vi "8HP_AVmod_EnFlo_Specific.vi"(2 "Datalog file path (full)":path, 3 "COM port":refnum<visa-resource-name>, 4 "Log data stream":bool, 5 "Set data rate (Hz)":u8(ring)=14 items=["1", "2", "4", "5", "8", "10", "16", "20", "25", "32", "40", "50", "64", "80", "100", "125", "160", "200", "250", "320", "400", "500", "625", "800", "1000"], 6 "N samples":u32=1000, 7 "Command":T2="D") -> (0 "Error":errorcluster, 1 "All samples out":sgl[][](array[numeric]))   [LabVIEW 2020]
uses:
  ctls/8HP_Cmd (USB).ctl
  Globals/Meas_global.vi
panel:
  in  "Main":T1(tab)
  out "Serial number":sgl
  out "Subsystems ok":bool[](array[boolean])
  out "Pressure sensor values in range":bool[](array[boolean])
  out "Pressure sensor temperatures in range":bool[](array[boolean])
  out "Pressure sensor EEPROM checksums ok":bool[](array[boolean])
  out "P_raw_Azero":sgl[](array[numeric])
  out "n":u16
  out "Auto zero progBar":u16(slide) caption="Collecting samples, please maintain dP = 0" scale=0.0..1000.0
  in  "EEPROM array 2":u16[](array[numeric])
  in  "EEPROM array":sgl[](array[numeric])
  out "Chk ok":bool
  out "EEPROM Checksum":u16 format="%04x"
  out "received":bool
  out "Returned data rate (Hz)":u16
  out "sent":bool
  out "frm err":u32
  out "chk err":u32
  in  "Stop Data":bool
  out "Relative humidity (%)":sgl
  out "Env. sensor die temperature (deg C)":sgl
  out "External thermistor 0 temperature (deg C)":sgl
  out "Atmospheric pressure (mbar)":sgl
  out "Checksum ok":bool
  out "Gyration vector (deg / s)":sgl[](array[numeric])
  out "Acceleration vector (g)":sgl[](array[numeric])
  out "Pressures":sgl[][](graph)
  out "Stream enabled":bool
  out "External thermistor 1 temperature (deg C)":sgl
  # "Paul Nathan 05/2019"
  # "Output array order:\nP0 (Pa)\n  |\nP7 (Pa)\nT0 (deg C)\nT1 (deg C)\nP_atmos (mbar)\nT_env (deg C)\nRH (%)\nax (g)\nay (g)\naz (g)\nwx (deg / s)\nwy (deg / s)\nwz (deg / s)"
  # "Environmental sensor present"
  # "Inertial sensor present"
  # "Accelerometer self test pass"
  # "Gyroscope self test pass"
  # "External thermistor 0 value in range"
  # "External thermistor 1 value in range"
  # "MCU EEPROM checksum ok"
  # "Pressure sensor 0 value in range"
  # "Pressure sensor 1 value in range"
  # "Pressure sensor 2 value in range"
  # "Pressure sensor 3 value in range"
  # "Pressure sensor 4 value in range"
  # "Pressure sensor 5 value in range"
  # "Pressure sensor 6 value in range"
  # "Pressure sensor 7 value in range"
  # "Pressure sensor 0 temperature in range"
  # "Pressure sensor 1 temperature in range"
  # "Pressure sensor 2 temperature in range"
  # "Pressure sensor 3 temperature in range"
  # "Pressure sensor 4 temperature in range"
  # "Pressure sensor 5 temperature in range"
  # "Pressure sensor 6 temperature in range"
  # "Pressure sensor 7 temperature in range"
  # "Pressure sensor 0 EEPROM checksum okay"
  # "Pressure sensor 1 EEPROM checksum okay"
  # "Pressure sensor 2 EEPROM checksum okay"
  # "Pressure sensor 3 EEPROM checksum okay"
  # "Pressure sensor 4 EEPROM checksum okay"
  # "Pressure sensor 5 EEPROM checksum okay"
  # "Pressure sensor 6 EEPROM checksum okay"
  # "Pressure sensor 7 EEPROM checksum okay"
  # "of 1000"
  # "P0 raw auto-zero"
  # "P1 raw auto-zero"
  # "P2 raw auto-zero"
  # "P3 raw auto-zero"
  # "P4 raw auto-zero"
  # "P5 raw auto-zero"
  # "P6 raw auto-zero"
  # "P7 raw auto-zero"
  # "Power-up defaults"
  # "Data rate (Hz)"
  # "TTL streaming"
  # "USB streaming"
  # "TTL stream contains full data"
  # "Accelerometer range mode"
  # "Gyroscope range mode"
  # "IMU rate mode"
  # "P0 raw auto-zero"
  # "P1 raw auto-zero"
  # "P2 raw auto-zero"
  # "P3 raw auto-zero"
  # "P4 raw auto-zero"
  # "P5 raw auto-zero"
  # "P6 raw auto-zero"
  # "P7 raw auto-zero"
  # "Atmospheric pressure offset (Pa)"
  # "External thermistor 0 temperature offset (deg C)"
  # "External thermistor 1 temperature offset (deg C)"
  # "Serial number"
  # "Baud rate (bps)"
  # "Accelerometer vector magnitude scale factor"
  # "Gyroscope x component offset (deg / s)"
  # "Gyroscope y component offset (deg / s)"
  # "Gyroscope z component offset (deg / s)"
  # "w_x"
  # "w_y"
  # "w_z"
  # "a_x"
  # "a_y"
  # "a_z"
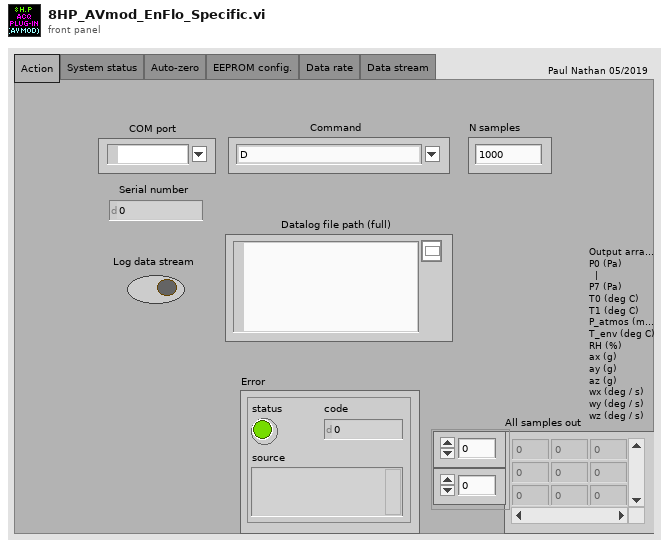
[diagram p1: front panel]
types:
  T1 = enum32{"Action", "System status", "Auto-zero", "EEPROM config.", "Data rate", "Data stream"}
  T2 = typedef "8HP_Cmd (USB).ctl" = string
  T3 = enum16{"open", "replace", "create", "open or create", "replace or create", "replace or create with confirmation"}
  T4 = typedef "Rendezvous RefNum" = refnum<k1>
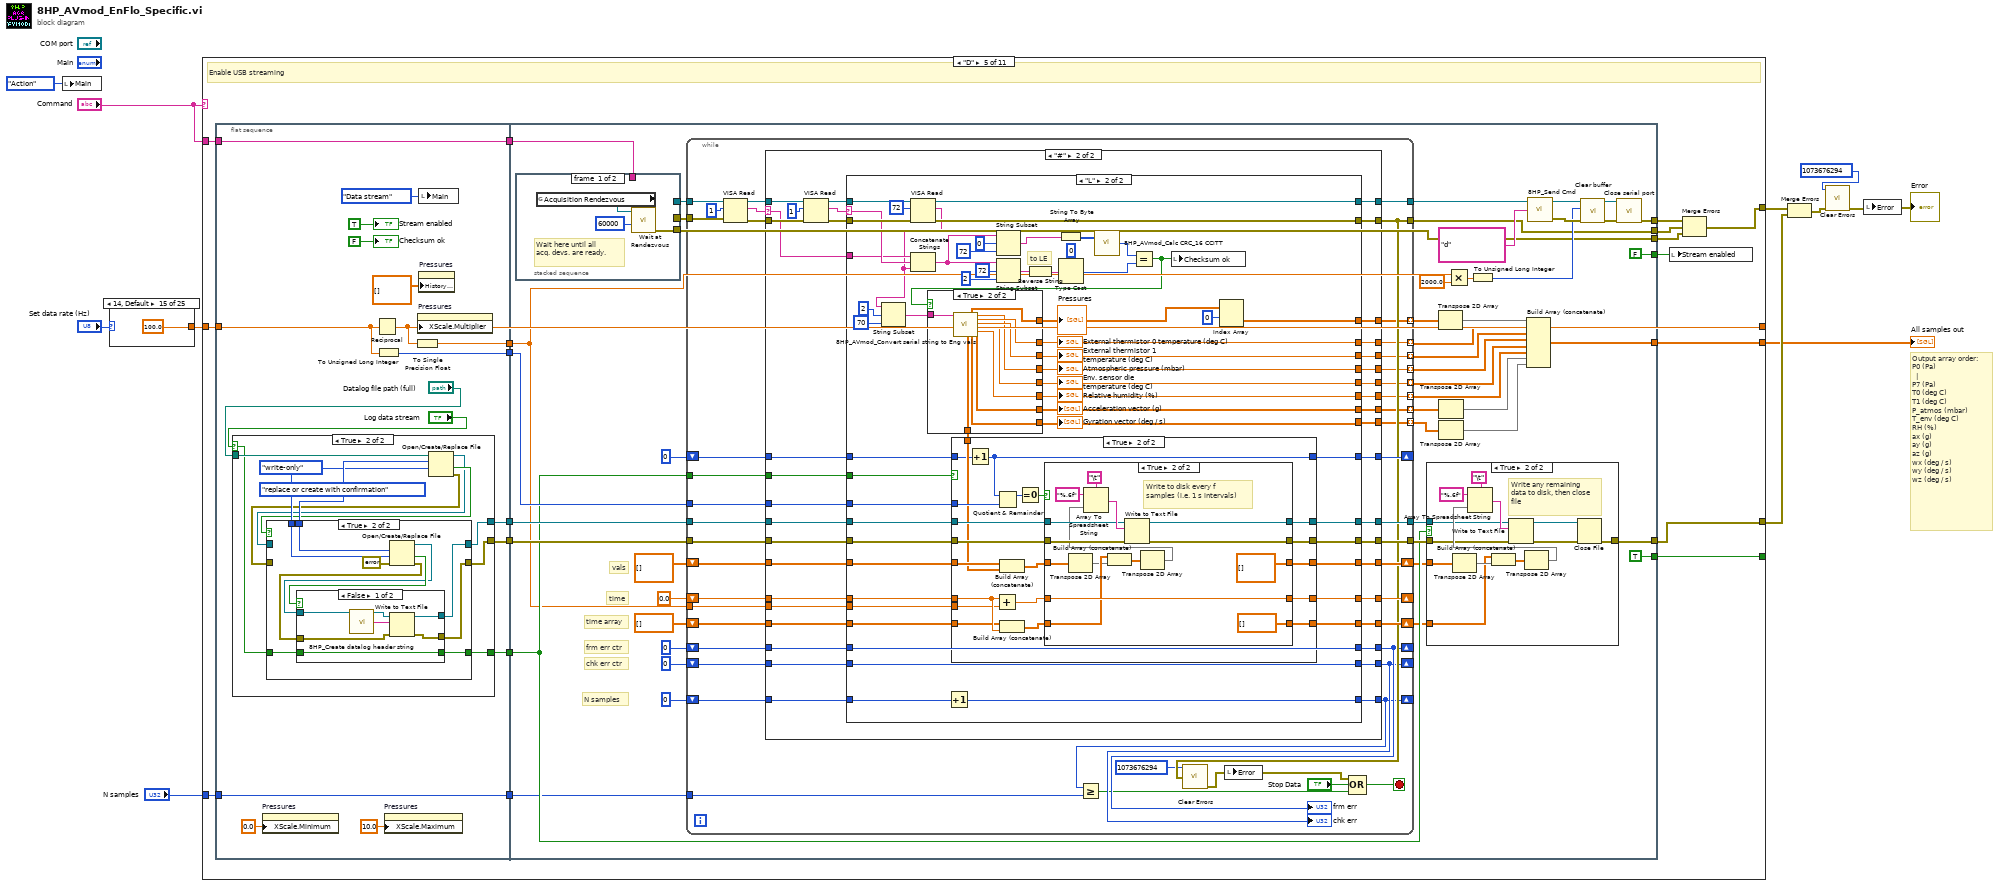
[diagram p0: block diagram]
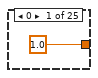
[diagram p2: hidden frame]
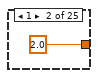
[diagram p3: hidden frame]
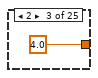
[diagram p4: hidden frame]
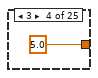
[diagram p5: hidden frame]
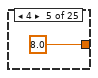
[diagram p6: hidden frame]
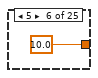
[diagram p7: hidden frame]
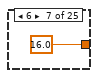
[diagram p8: hidden frame]
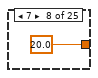
[diagram p9: hidden frame]
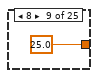
[diagram p10: hidden frame]
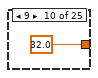
[diagram p11: hidden frame]
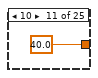
[diagram p12: hidden frame]
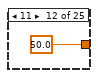
[diagram p13: hidden frame]
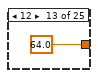
[diagram p14: hidden frame]
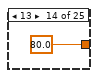
[diagram p15: hidden frame]
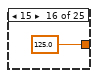
[diagram p16: hidden frame]
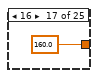
[diagram p17: hidden frame]
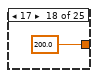
[diagram p18: hidden frame]
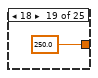
[diagram p19: hidden frame]
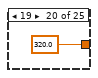
[diagram p20: hidden frame]
diagram:
  # "Output array order:\nP0 (Pa)\n  |\nP7 (Pa)\nT0 (deg C)\nT1 (deg C)\nP_atmos (mbar)\nT_env (deg C)\nRH (%)\nax (g)\nay (g)\naz (g)\nwx (deg / s)\nwy (deg / s)\nwz (deg / s)"
  n1 = local write "Main"(T1."Action" ("Main")) -> ()
  n2 = case shown="14, Default" "Set data rate (Hz)" {
    tunnel: [1.0 2.0 4.0 5.0 8.0 10.0 16.0 20.0 25.0 32.0 40.0 50.0 64.0 80.0 100.0 125.0 160.0 200.0 250.0 320.0 400.0 500.0 625.0 800.0 1000.0] -> w6
    frame 0 {
    }
    frame 1 {
    }
    frame 2 {
    }
    frame 3 {
    }
    frame 4 {
    }
    frame 5 {
    }
    frame 6 {
    }
    frame 7 {
    }
    frame 8 {
    }
    frame 9 {
    }
    frame 10 {
    }
    frame 11 {
    }
    frame 12 {
    }
    frame 13 {
    }
    frame 14, Default {
    }
    frame 15 {
    }
    frame 16 {
    }
    frame 17 {
    }
    frame 18 {
    }
    frame 19 {
    }
    frame 20 {
    }
    frame 21 {
    }
    frame 22 {
    }
    frame 23 {
    }
    frame 24 {
    }
  }
  n3 = case shown="\"D\"" "Command" {
    tunnel: [w41 w80 w117 w186 w277 w631 w655 w711 w747 FALSE FALSE] -> _
    tunnel: "Command" -> [w40 w79 w116 w197 w276 w633 w661 w717 w746 _ _]
    tunnel: [w38 w77 w114 w190 w264 w632 w656 w712 w744 errorcluster {"status"=FALSE, "code"=0, "source"=""} ("Error out") errorcluster {"status"=FALSE, "code"=0, "source"=""} ("Error out")] -> w10
    tunnel: [_ _ _ _ w274 _ _ _ _ _ _] -> w9
    tunnel: w6 -> [w37 w76 w113 w194 w267 w629 _ _ w743 w767 w770]
    tunnel: [w37 w76 w113 w194 w267 w629 w657 w713 w743 w767 w770] -> _
    tunnel: "N samples" -> [_ _ _ _ w262 _ _ _ _ _ _]
    tunnel: [_ _ _ _ w261 _ _ _ _ _ _] -> w3
    frame "S", "s" {
      # "Perform self-test and retrieve status bytes, Retrieve status bytes"
      n4 = flat-sequence {
        tunnel: w40 -> [w44]
        tunnel: [w44] -> w39
        tunnel: [TRUE] -> w41
        tunnel: w39 -> [w50]
        tunnel: [w45] -> w38
        frame #0 {
          w43 = bool[] [] ("Pressure sensor EEPROM checksums ok")
          n5 = local write "Main"(T1."System status" ("Main")) -> ()
          "Pressure sensor EEPROM checksums ok" <- w43
          "Pressure sensor temperatures in range" <- w43
          "Pressure sensor values in range" <- w43
          "Subsystems ok" <- w43
        }
        frame #1 {
          w55 = 1 ("length (rest)")
          w63 = u8 0 ("byte count")
          n6 = local read "COM port"() -> (w51:refnum<visa-resource-name>)
          n7 = call "Open serial port.vi"("timeout (ms)"=u32 5000, "VISA resource name"=w51) -> ("Error out"=w73:errorcluster, "VISA resource name out"=w74:refnum<visa-resource-name>)  [unwired: 8 in]
          n8 = call "8HP_Send Cmd.vi"("Error In"=w73, "Operation"=w50, "Port"=w74) -> ("Error Out"=w71:errorcluster, "Port out"=w72:refnum<visa-resource-name>)  [unwired: 1 in]
          n9 = VISA Read(VISA resource name=w72, byte count=u32 4, error in (no error)=w71) -> (VISA resource name out=w69:refnum<visa-resource-name>, read buffer=w58:string, error out=w68:errorcluster)  [unwired: 1 out]
          n10 = call "Close serial port.vi"("Error in"=w68, "VISA resource name"=w69) -> ("Error out"=w45:errorcluster)  [unwired: 9 in]
          n11 = String Subset(string=w58, offset (0)=0, length (rest)=w55) -> (substring=w67:string)
          n12 = String Subset(string=w58, offset (0)=1, length (rest)=w55) -> (substring=w66:string)
          n13 = String Subset(string=w58, offset (0)=2 ("length (rest)"), length (rest)=w55) -> (substring=w65:string)
          n14 = String Subset(string=w58, offset (0)=3, length (rest)=w55) -> (substring=w64:string)
          n15 = Type Cast(type=w63, x=w67) -> (*(type *) &x=w62:u8)
          n16 = Type Cast(type=w63, x=w66) -> (*(type *) &x=w61:u8)
          n17 = Type Cast(type=w63, x=w65) -> (*(type *) &x=w60:u8)
          n18 = Type Cast(type=w63, x=w64) -> (*(type *) &x=w59:u8)
          n19 = Number To Boolean Array(number=w62) -> (Boolean array=w49:bool[])
          n20 = Number To Boolean Array(number=w61) -> (Boolean array=w48:bool[])
          n21 = Number To Boolean Array(number=w60) -> (Boolean array=w47:bool[])
          n22 = Number To Boolean Array(number=w59) -> (Boolean array=w46:bool[])
          n23 = local write "Pressure sensor EEPROM checksums ok"(w49) -> ()
          n24 = local write "Pressure sensor temperatures in range"(w48) -> ()
          n25 = local write "Pressure sensor values in range"(w47) -> ()
          n26 = local write "Subsystems ok"(w46) -> ()
        }
      }
    }
    frame "Z", "z" {
      # "Perform permanent auto-zero (write values to EEPROM), Perform temporary auto-zero"
      n27 = flat-sequence {
        tunnel: w79 -> [w84]
        tunnel: [w84] -> w78
        tunnel: [TRUE] -> w80
        tunnel: w78 -> [w91]
        tunnel: [w87] -> w77
        frame #0 {
          n28 = local write "Main"(T1."Auto-zero" ("Main")) -> ()
          "P_raw_Azero" <- sgl[] [] ("P_raw_Azero")
          "Auto zero progBar" <- u16 0 ("Collecting samples, please maintain dP = 0")
        }
        frame #1 {
          n29 = local read "COM port"() -> (w92:refnum<visa-resource-name>)
          n30 = call "Open serial port.vi"("timeout (ms)"=u32 16000, "VISA resource name"=w92) -> ("Error out"=w99:errorcluster, "VISA resource name out"=w100:refnum<visa-resource-name>)  [unwired: 8 in]
          n31 = call "8HP_Send Cmd.vi"("Error In"=w99, "Operation"=w91, "Port"=w100) -> ("Error Out"=w97:errorcluster, "Port out"=w98:refnum<visa-resource-name>)  [unwired: 1 in]
          n32 = VISA Read(VISA resource name=w98, byte count=u32 32, error in (no error)=w97) -> (VISA resource name out=w95:refnum<visa-resource-name>, read buffer=w88:string, error out=w94:errorcluster)  [unwired: 1 out]
          n33 = for {
            N: 1000 -> [_]
            shift-right: [w102] -> _
            shift-left: u16 0 -> [w103]
            n34 = Increment(x=w103) -> (x+1=w102:u16)
            "n" <- w102
            n35 = Wait (ms)(milliseconds to wait=u32 10) -> ()  [unwired: 1 out]
            n36 = local write "Auto zero progBar"(w102) -> ()
          }
          n37 = for {
            N: 8 -> [_]
            tunnel: [w106] -> w90 mode=indexing
            tunnel: w88 -> [w105]
            i -> [w112]
            w110 = 4 ("x")
            # "to BE"
            n38 = Multiply(x=w110, y=w112) -> (x*y=w111:i32)
            n39 = String Subset(string=w105, offset (0)=w111, length (rest)=w110) -> (substring=w109:string)
            n40 = Reverse String(1:w109) -> (0:w108:string)
            n41 = Type Cast(type=sgl 0.0 ("byte count"), x=w108) -> (*(type *) &x=w106:sgl)
          }
          n42 = call "Close serial port.vi"("Error in"=w94, "VISA resource name"=w95) -> ("Error out"=w87:errorcluster)  [unwired: 9 in]
          n43 = local write "P_raw_Azero"(w90) -> ()
        }
      }
    }
    frame "R" {
      # "Read all EEPROM values"
      n44 = flat-sequence {
        tunnel: w116 -> [w121]
        tunnel: [w121] -> w115
        tunnel: [TRUE] -> w117
        tunnel: w115 -> [w159]
        tunnel: [w157] -> w114
        frame #0 {
          n45 = local write "EEPROM array"(sgl[] [] ("EEPROM array")) -> ()
          n46 = local write "EEPROM array 2"(u16[] [] ("EEPROM array 2")) -> ()
          n47 = local write "Main"(T1."EEPROM config." ("Main")) -> ()
        }
        frame #1 {
          # "to BE"
          # "to BE"
          n48 = local read "COM port"() -> (w160:refnum<visa-resource-name>)
          n49 = call "Open serial port.vi"("timeout (ms)"=u32 5000, "VISA resource name"=w160) -> ("Error out"=w167:errorcluster, "VISA resource name out"=w168:refnum<visa-resource-name>)  [unwired: 8 in]
          n50 = call "8HP_Send Cmd.vi"("Error In"=w167, "Operation"=w159, "Port"=w168) -> ("Error Out"=w165:errorcluster, "Port out"=w166:refnum<visa-resource-name>)  [unwired: 1 in]
          n51 = VISA Read(VISA resource name=w166, byte count=u32 78, error in (no error)=w165) -> (VISA resource name out=w163:refnum<visa-resource-name>, read buffer=w126:string, error out=w162:errorcluster)  [unwired: 1 out]
          n52 = call "Close serial port.vi"("Error in"=w162, "VISA resource name"=w163) -> ("Error out"=w157:errorcluster)  [unwired: 9 in]
          n53 = String Subset(string=w126, offset (0)=0, length (rest)=56 ("length (rest)")) -> (substring=w155:string)
          n54 = String Subset(string=w126, offset (0)=64, length (rest)=12 ("length (rest)")) -> (substring=w150:string)
          n55 = String Subset(string=w126, offset (0)=56, length (rest)=2 ("length (rest)")) -> (substring=w140:string)
          n56 = String Subset(string=w126, offset (0)=58, length (rest)=6 ("length (rest)")) -> (substring=w135:string)
          n57 = String Subset(string=w126, offset (0)=76, length (rest)=2 ("length (rest)")) -> (substring=w127:string)
          n58 = String Subset(string=w126, offset (0)=0, length (rest)=76 ("length (rest)")) -> (substring=w123:string)
          n59 = for {
            N: 14 -> [_]
            tunnel: [w181] -> w149 mode=indexing
            tunnel: w155 -> [w180]
            i -> [w185]
            w183 = 4 ("x")
            # "to BE"
            n60 = Multiply(x=w183, y=w185) -> (x*y=w184:i32)
            n61 = String Subset(string=w180, offset (0)=w184, length (rest)=w183) -> (substring=w179:string)
            n62 = Reverse String(1:w179) -> (0:w178:string)
            n63 = Type Cast(type=sgl 0.0 ("byte count"), x=w178) -> (*(type *) &x=w181:sgl)
          }
          n64 = for {
            N: 3 -> [_]
            tunnel: [w173] -> w148 mode=indexing
            tunnel: w150 -> [w172]
            i -> [w177]
            w175 = 4 ("x")
            # "to BE"
            n65 = Multiply(x=w175, y=w177) -> (x*y=w176:i32)
            n66 = String Subset(string=w172, offset (0)=w176, length (rest)=w175) -> (substring=w171:string)
            n67 = Reverse String(1:w171) -> (0:w170:string)
            n68 = Type Cast(type=sgl 0.0 ("byte count"), x=w170) -> (*(type *) &x=w173:sgl)
          }
          n69 = Reverse String(1:w140) -> (0:w146:string)
          n70 = Reverse String(1:w127) -> (0:w131:string)
          n71 = String To Byte Array(string=w123) -> (unsigned byte array=w134:u8[])
          n72 = call "8HP_AVmod_Calc CRC_16 CCITT.vi"("Data bytes"=w134) -> ("CRC_16-CCITT"=w133:u16)  [unwired: 1 in]
          n73 = Type Cast(type=u16 0 ("byte count"), x=w146) -> (*(type *) &x=w139:u16)
          n74 = Type Cast(type=u16 0 ("byte count"), x=w131) -> (*(type *) &x=w122:u16)
          n75 = String To Byte Array(string=w135) -> (unsigned byte array=w138:u8[])
          n76 = To Unsigned Word Integer(number=w138) -> (unsigned 16bit integer=w136:u16[])
          n77 = Equal?(x=w122, y=w133) -> (x = y?=w132:bool)
          n78 = Build Array (concatenate)(w149, w148) -> (w147:sgl[])
          n79 = Build Array (concatenate)(w139, w136) -> (w137:u16[])
          n80 = local write "EEPROM array"(w147) -> ()
          n81 = local write "EEPROM array 2"(w137) -> ()
          n82 = local write "EEPROM Checksum"(w122) -> ()
          n83 = local write "Chk ok"(w132) -> ()
        }
      }
    }
    frame "W" {
      # "Write all EEPROM values (including new checksum)"
      n84 = flat-sequence {
        tunnel: w197 -> [w216]
        tunnel: [w216] -> w196
        tunnel: [w210] -> w195
        tunnel: [w209] -> w193
        tunnel: [w205] -> w192
        tunnel: [w206] -> w191
        tunnel: [TRUE] -> w187
        tunnel: w196 -> [w242]
        tunnel: w195 -> [w237]
        tunnel: [w236] -> w190
        tunnel: w193 -> [w228]
        tunnel: w192 -> [w225]
        tunnel: w191 -> [w223]
        frame #0 {
          n85 = local write "Main"(T1."EEPROM config." ("Main")) -> ()
          n86 = Split 1D Array(array="EEPROM array", index=14) -> (first subarray=w210:sgl[], second subarray=w209:sgl[])
          n87 = Split 1D Array(array="EEPROM array 2", index=1) -> (first subarray=w208:u16[], second subarray=w207:u16[])
          n88 = Index Array(array=w208, index=0) -> (element=w205:u16)
          n89 = To Unsigned Byte Integer(number=w207) -> (unsigned 8bit integer=w206:u8[])
        }
        frame #1 {
          # "to LE"
          # "to LE"
          n90 = local read "COM port"() -> (w243:refnum<visa-resource-name>)
          n91 = for {
            N: 14 -> [_]
            tunnel: w237 -> [w256] mode=indexing
            shift-right: [w257] -> w232
            shift-left: "" -> [w258]
            # "to LE"
            n92 = Type Cast(type="", x=w256) -> (*(type *) &x=w255:string)
            n93 = Reverse String(1:w255) -> (0:w254:string)
            n94 = Concatenate Strings(w258, w254) -> (w257:string)
          }
          n95 = for {
            N: 3 -> [_]
            tunnel: w228 -> [w250] mode=indexing
            shift-right: [w251] -> w222
            shift-left: "" -> [w252]
            # "to LE"
            n96 = Type Cast(type="", x=w250) -> (*(type *) &x=w249:string)
            n97 = Reverse String(1:w249) -> (0:w248:string)
            n98 = Concatenate Strings(w252, w248) -> (w251:string)
          }
          n99 = Type Cast(type="", x=w225) -> (*(type *) &x=w227:string)
          n100 = Reverse String(1:w227) -> (0:w224:string)
          n101 = Byte Array To String(unsigned byte array=w223) -> (string=w221:string)
          n102 = call "Open serial port.vi"("timeout (ms)"=u32 5000, "VISA resource name"=w243) -> ("Error out"=w245:errorcluster, "VISA resource name out"=w246:refnum<visa-resource-name>)  [unwired: 8 in]
          n103 = Concatenate Strings(w232, w224, w221, w222) -> (w231:string)
          n104 = String To Byte Array(string=w231) -> (unsigned byte array=w220:u8[])
          n105 = call "8HP_AVmod_Calc CRC_16 CCITT.vi"("Data bytes"=w220) -> ("CRC_16-CCITT"=w219:u16)  [unwired: 1 in]
          "EEPROM Checksum" <- w219
          n106 = Type Cast(type="", x=w219) -> (*(type *) &x=w218:string)
          n107 = Reverse String(1:w218) -> (0:w217:string)
          n108 = Concatenate Strings(w231, w217) -> (w235:string)
          n109 = call "8HP_Send Cmd + Data.vi"("Error In"=w245, "Data"=w235, "Operation"=w242, "Port"=w246) -> ("Error Out"=w233:errorcluster, "Port out"=w234:refnum<visa-resource-name>)  [unwired: 1 in]
          n110 = call "Close serial port.vi"("Error in"=w233, "VISA resource name"=w234) -> ("Error out"=w236:errorcluster)  [unwired: 9 in]
          "Chk ok" <- TRUE ("Chk ok")
        }
      }
      n111 = flat-sequence {
        tunnel: [w198] -> w188
        tunnel: w187 -> [w198]
        tunnel: [w200] -> w189
        tunnel: w188 -> [w200]
        tunnel: [w202] -> w186
        tunnel: w189 -> [w202]
        frame #0 {
          n112 = local write "Main"(T1."Action" ("Main")) -> ()
        }
        frame #1 {
          n113 = One Button Dialog(message="Application restart required after making changes to the EEPROM.\nThe application will now exit. Please re-run.") -> ()  [unwired: 1 in, 1 out]
        }
        frame #2 {
          n114 = Stop(stop? (T)=TRUE) -> ()
        }
      }
    }
    frame "D" {
      # "Enable USB streaming"
      n115 = flat-sequence {
        tunnel: w276 -> [w294]
        tunnel: [w294] -> w275
        tunnel: [w291] -> w273
        tunnel: [w290] -> w272
        tunnel: [w289] -> w271
        tunnel: w267 -> [w281]
        tunnel: [w287] -> w270
        tunnel: [w283] -> w269
        tunnel: [w278] -> w263
        tunnel: w262 -> [w278]
        tunnel: [TRUE] -> w277
        tunnel: w275 -> [w352]
        tunnel: [w378] -> w265
        tunnel: [w377] -> w274
        tunnel: w273 -> [w374]
        tunnel: w272 -> [w373]
        tunnel: w271 -> [w375]
        tunnel: w270 -> [w346]
        tunnel: w269 -> [w367]
        tunnel: [FALSE] -> w268
        tunnel: [w351] -> w266
        tunnel: w263 -> [w348]
        tunnel: [w334] -> w261
        tunnel: [w333] -> w260
        frame #0 {
          n116 = case shown="True" "Log data stream" {
            selector: "Log data stream" -> [w295 w298]
            tunnel: "Datalog file path (full)" -> [_ w307]
            tunnel: [refnum<file> refnum ("refnum out") w304] -> w291
            tunnel: [errorcluster {"status"=FALSE, "code"=0, "source"=""} ("error out") w303] -> w290
            tunnel: [w295 w299] -> w283
            frame False {
            }
            frame True {
              w305 = enum16{"read/write", "read-only", "write-only"}."write-only" ("access (0:read/write)")
              w306 = T3."replace or create with confirmation" ("operation (0:open)")
              n117 = Open/Create/Replace File(file path (use dialog)=w307, operation (0:open)=w306, access (0:read/write)=w305) -> (refnum out=w300:refnum<file>, cancelled=w302:bool, error out=w301:errorcluster)  [unwired: 3 in]
              n118 = case shown="True" w302 {
                tunnel: w306 -> [_ w323]
                tunnel: w305 -> [_ w322]
                tunnel: w301 -> [w311 _]
                tunnel: [w309 w317] -> w304
                tunnel: [w310 w318] -> w303
                tunnel: w300 -> [w312 _]
                tunnel: [w308 w315] -> w299
                tunnel: w298 -> [w308 w314]
                frame False {
                  n119 = call "8HP_Create datalog header string.vi"() -> ("Datalog header string"=w313:string)  [unwired: 1 in]
                  n120 = Write to Text File(file (use dialog)=w312, text=w313, error in=w311) -> (refnum out=w309:refnum<file>, error out=w310:errorcluster)  [unwired: 1 in, 1 out]
                }
                frame True {
                  n121 = Open/Create/Replace File(error in=errorcluster {"status"=FALSE, "code"=0, "source"=""}, operation (0:open)=w323, access (0:read/write)=w322) -> (refnum out=w320:refnum<file>, cancelled=w321:bool, error out=w319:errorcluster)  [unwired: 3 in]
                  n122 = case shown="False" w321 {
                    tunnel: w320 -> [w328 _]
                    tunnel: w319 -> [w327 _]
                    tunnel: [w326 errorcluster {"status"=FALSE, "code"=0, "source"=""} ("error out")] -> w318
                    tunnel: [w325 refnum<file> refnum ("t")] -> w317
                    tunnel: [w324 w330] -> w315
                    tunnel: w314 -> [w324 _]
                    frame False {
                      n123 = call "8HP_Create datalog header string.vi"() -> ("Datalog header string"=w329:string)  [unwired: 1 in]
                      n124 = Write to Text File(file (use dialog)=w328, text=w329, error in=w327) -> (refnum out=w325:refnum<file>, error out=w326:errorcluster)  [unwired: 1 in, 1 out]
                    }
                    frame True {
                      w330 = FALSE ("Log data stream")
                      n125 = local write "Log data stream"(w330) -> ()
                    }
                  }
                }
              }
            }
          }
          n126 = property on="Pressures" class="WFChart (strict)"("XScale.Minimum"=0.0 ("X Scale.Range:Minimum")) -> ()  [unwired: 2 in, 2 out]
          n127 = Reciprocal(x=w281) -> (1/x=w288:dbl)
          n128 = To Unsigned Long Integer(number=w281) -> (unsigned 32bit integer=w289:u32)
          n129 = property on="Pressures" class="WFChart (strict)"("XScale.Maximum"=10.0 ("X Scale.Range:Minimum")) -> ()  [unwired: 2 in, 2 out]
          n130 = To Single Precision Float(number=w288) -> (single precision float=w287:sgl)
          n131 = property on="Pressures" class="WFChart (strict)"("XScale.Multiplier"=w288) -> ()  [unwired: 2 in, 2 out]
          n132 = local write "Main"(T1."Data stream" ("Main")) -> ()
          n133 = property on="Pressures" class="WFChart (strict)"("History Data"=sgl[][] []) -> ()  [unwired: 2 in, 2 out]
          "Checksum ok" <- FALSE ("Checksum ok")
          "Stream enabled" <- TRUE ("Stream enabled")
        }
        frame #1 {
          # "N samples"
          # "chk err ctr"
          # "frm err ctr"
          # "vals"
          # "time"
          # "time array"
          n134 = stacked-sequence {
            tunnel: [_ w387] -> w366
            tunnel: [_ w385] -> w365
            tunnel: w352 -> [_ w383]
            tunnel: [w380 _] -> w333
            frame #0 {
              # "Wait here until all acq. devs. are ready."
              n135 = global read "Meas_global.vi" "Acquisition Rendezvous"() -> (w382:T4)
              n136 = call <vilib>:"Wait at Rendezvous.vi"("ms timeout (-1)"=60000, "rendezvous"=w382) -> ("error out"=w380:errorcluster)  [unwired: 3 in, 2 out]
            }
            frame #1 {
              n137 = local read "COM port"() -> (w389:refnum<visa-resource-name>)
              n138 = call "Open serial port.vi"("timeout (ms)"=u32 5000, "VISA resource name"=w389) -> ("Error out"=w386:errorcluster, "VISA resource name out"=w388:refnum<visa-resource-name>)  [unwired: 8 in]
              n139 = call "8HP_Send Cmd.vi"("Error In"=w386, "Operation"=w383, "Port"=w388) -> ("Error Out"=w385:errorcluster, "Port out"=w387:refnum<visa-resource-name>)  [unwired: 1 in]
            }
          }
          n140 = while {
            tunnel: [w408] -> w351
            tunnel: w366 -> [w410]
            tunnel: [w428] -> w364
            shift-right: [w424] -> _
            shift-left: u32 0 -> [w425]
            tunnel: w375 -> [w423]
            tunnel: w374 -> [w422]
            tunnel: w373 -> [w421]
            tunnel: [w420] -> w372
            tunnel: [w419] -> w371
            shift-right: [w418] -> w355
            shift-left: sgl[][] [] -> [w417]
            shift-right: [w414] -> _
            shift-left: sgl 0.0 ("Numeric") -> [w416]
            tunnel: w346 -> [w415]
            shift-right: [w412] -> w354
            shift-left: sgl[] [] -> [w413]
            tunnel: w367 -> [w411]
            tunnel: w365 -> [w409]
            shift-right: [w403] -> _
            shift-left: u32 0 -> [w405]
            shift-right: [w402] -> _
            shift-left: u32 0 -> [w404]
            tunnel: w348 -> [w399]
            shift-right: [w398] -> _
            shift-left: u32 0 -> [w401]
            tunnel: [w397] -> w342 mode=indexing
            tunnel: [w396] -> w341 mode=indexing
            tunnel: [w395] -> w340 mode=indexing
            tunnel: [w394] -> w339 mode=indexing
            tunnel: [w393] -> w338 mode=indexing
            tunnel: [w392] -> w337 mode=indexing
            tunnel: [w391] -> w336 mode=indexing
            tunnel: [w390] -> w335 mode=indexing
            stop <- w426 stop-if-true
            n141 = VISA Read(VISA resource name=w410, byte count=u32 1, error in (no error)=w409) -> (VISA resource name out=w430:refnum<visa-resource-name>, read buffer=w431:string, error out=w429:errorcluster)  [unwired: 1 out]
            n142 = case shown="\"#\"" w431 {
              selector: w431 -> [_ w455]
              tunnel: w430 -> [w443 w460]
              tunnel: [w444 w481] -> w408
              tunnel: w429 -> [w444 w459]
              tunnel: [w443 w482] -> w428
              tunnel: w425 -> [w442 w480]
              tunnel: [w442 w479] -> w424
              tunnel: w423 -> [_ w478]
              tunnel: w422 -> [w441 w477]
              tunnel: w421 -> [w440 w476]
              tunnel: [w440 w475] -> w420
              tunnel: [w441 w474] -> w419
              tunnel: [w439 w473] -> w418
              tunnel: w417 -> [w439 w472]
              tunnel: w416 -> [w438 w471]
              tunnel: w415 -> [_ w470]
              tunnel: [w438 w469] -> w414
              tunnel: w413 -> [w437 w468]
              tunnel: [w437 w467] -> w412
              tunnel: w411 -> [_ w466]
              tunnel: w405 -> [w436 w465]
              tunnel: w404 -> [w435 w464]
              tunnel: [w434 w463] -> w403
              tunnel: [w435 w462] -> w402
              tunnel: w401 -> [w433 w454]
              tunnel: [w433 w453] -> w398
              tunnel: [_ w452] -> w397
              tunnel: [_ w451] -> w396
              tunnel: [_ w450] -> w395
              tunnel: [_ w449] -> w394
              tunnel: [_ w448] -> w393
              tunnel: [_ w447] -> w392
              tunnel: [_ w446] -> w391
              tunnel: [_ w445] -> w390
              frame Default {
                # "Frame error"
                n143 = Increment(x=w436) -> (x+1=w434:u32)
              }
              frame "#" {
                n144 = VISA Read(VISA resource name=w460, byte count=u32 1, error in (no error)=w459) -> (VISA resource name out=w458:refnum<visa-resource-name>, read buffer=w456:string, error out=w457:errorcluster)  [unwired: 1 out]
                n145 = case shown="\"L\"" w456 {
                  selector: w456 -> [_ w526]
                  tunnel: w457 -> [w493 w548]
                  tunnel: w458 -> [w494 w547]
                  tunnel: [w494 w546] -> w482
                  tunnel: [w493 w545] -> w481
                  tunnel: w480 -> [w484 w543]
                  tunnel: [w484 w542] -> w479
                  tunnel: w478 -> [_ w541]
                  tunnel: w477 -> [w485 w540]
                  tunnel: w476 -> [w486 w539]
                  tunnel: [w486 w538] -> w475
                  tunnel: [w485 w537] -> w474
                  tunnel: [w487 w536] -> w473
                  tunnel: w472 -> [w487 w535]
                  tunnel: w471 -> [w488 w534]
                  tunnel: w470 -> [_ w533]
                  tunnel: [w488 w532] -> w469
                  tunnel: w468 -> [w489 w531]
                  tunnel: [w489 w530] -> w467
                  tunnel: w466 -> [_ w529]
                  tunnel: w465 -> [w492 w528]
                  tunnel: w464 -> [w490 w527]
                  tunnel: [w491 w528] -> w463
                  tunnel: [w490 w527] -> w462
                  tunnel: w455 -> [_ w525]
                  tunnel: w454 -> [w483 w508]
                  tunnel: [w483 w507] -> w453
                  tunnel: [_ w502] -> w452
                  tunnel: [_ w501] -> w451
                  tunnel: [_ w500] -> w450
                  tunnel: [_ w499] -> w449
                  tunnel: [_ w498] -> w448
                  tunnel: [_ w497] -> w447
                  tunnel: [_ w496] -> w446
                  tunnel: [_ w495] -> w445
                  frame Default {
                    n146 = Increment(x=w492) -> (x+1=w491:u32)
                  }
                  frame "L" {
                    # "to LE"
                    n147 = VISA Read(VISA resource name=w547, byte count=u32 72, error in (no error)=w548) -> (VISA resource name out=w546:refnum<visa-resource-name>, read buffer=w521:string, error out=w545:errorcluster)  [unwired: 1 out]
                    n148 = String Subset(string=w521, offset (0)=2, length (rest)=70 ("length (rest)")) -> (substring=w523:string)
                    n149 = Concatenate Strings(w525, w526, w521) -> (w510:string)
                    n150 = Increment(x=w508) -> (x+1=w507:u32)
                    n151 = String Subset(string=w510, offset (0)=0, length (rest)=72 ("length (rest)")) -> (substring=w509:string)
                    n152 = String Subset(string=w510, offset (0)=72, length (rest)=2 ("length (rest)")) -> (substring=w516:string)
                    n153 = Reverse String(1:w516) -> (0:w515:string)
                    n154 = String To Byte Array(string=w509) -> (unsigned byte array=w520:u8[])
                    n155 = Type Cast(type=u16 0 ("length (rest)"), x=w515) -> (*(type *) &x=w514:u16)
                    n156 = call "8HP_AVmod_Calc CRC_16 CCITT.vi"("Data bytes"=w520) -> ("CRC_16-CCITT"=w513:u16)  [unwired: 1 in]
                    n157 = Equal?(x=w513, y=w514) -> (x = y?=w505:bool)
                    n158 = case shown="True" w505 {
                      tunnel: w523 -> [_ w568]
                      tunnel: [w552 w567] -> w503
                      tunnel: [w551 w566] -> w501
                      tunnel: [w551 w565] -> w500
                      tunnel: [w551 w564] -> w498
                      tunnel: [w551 w563] -> w497
                      tunnel: [w550 w562] -> w496
                      tunnel: [w550 w561] -> w495
                      tunnel: [w549 w560] -> w506
                      tunnel: [w551 w559] -> w499
                      frame False {
                        (unwired) 3 ("dimension size")
                        w551 = sgl nan ("Atmospheric pressure (mbar)")
                        n159 = Initialize Array(sgl nan ("element"), 8 ("dimension size")) -> (w556:sgl[])
                        n160 = Initialize Array(sgl nan ("element")) -> (w550:sgl[])  [unwired: 1 in]
                        n161 = Initialize Array(sgl nan ("element"), 19 ("dimension size")) -> (w549:sgl[])
                        n162 = Build Array(w556) -> (w552:sgl[][])
                      }
                      frame True {
                        n163 = call "8HP_AVmod_Convert serial string to Eng vals.vi"("Serial buffer string (excluding FrameChars and MsgLen word)"=w568) -> ("All vals"=w560:sgl[], "Pressures"=w567:sgl[][], "Gyration vector (deg / s)"=w561:sgl[], "Atmospheric pressure (mbar)"=w559:sgl, "External thermistor 0 temperature (deg C)"=w566:sgl, "External thermistor 1 temperature (deg C)"=w565:sgl, "Env. sensor die temperature (deg C)"=w564:sgl, "Relative humidity (%)"=w563:sgl, "Acceleration vector (g)"=w562:sgl[])  [unwired: 10 in]
                      }
                    }
                    "Pressures" <- w503
                    "Acceleration vector (g)" <- w496
                    "Gyration vector (deg / s)" <- w495
                    "Atmospheric pressure (mbar)" <- w499
                    "External thermistor 0 temperature (deg C)" <- w501
                    "Env. sensor die temperature (deg C)" <- w498
                    "Relative humidity (%)" <- w497
                    "External thermistor 1 temperature (deg C)" <- w500
                    n164 = case shown="True" w529 {
                      tunnel: w543 -> [w574 w576]
                      tunnel: [w574 w575] -> w542
                      tunnel: w541 -> [_ w594]
                      tunnel: w506 -> [_ w580]
                      tunnel: w540 -> [w572 w591]
                      tunnel: w539 -> [w573 w590]
                      tunnel: [w573 w589] -> w538
                      tunnel: [w572 w588] -> w537
                      tunnel: w535 -> [w571 w581]
                      tunnel: [w571 w587] -> w536
                      tunnel: w534 -> [w570 w584]
                      tunnel: w533 -> [_ w583]
                      tunnel: [w570 w586] -> w532
                      tunnel: w531 -> [w569 w582]
                      tunnel: [w569 w585] -> w530
                      frame False {
                      }
                      frame True {
                        n165 = Increment(x=w576) -> (x+1=w575:u32)
                        n166 = Add(x=w584, y=w583) -> (x+y=w579:sgl)
                        n167 = Quotient & Remainder(x=w575, y=w594) -> (x-y*floor(x/y)=w593:u32)  [unwired: 1 out]
                        n168 = Build Array (concatenate)(w581, w580) -> (w577:sgl[][])
                        n169 = Build Array (concatenate)(w582, w584) -> (w578:sgl[])
                        n170 = Equal To 0?(x=w593) -> (x = 0?=w592:bool)
                        n171 = case shown="True" w592 {
                          tunnel: w591 -> [w598 w611]
                          tunnel: w590 -> [w599 w610]
                          tunnel: [w599 w609] -> w589
                          tunnel: [w598 w608] -> w588
                          tunnel: w577 -> [w596 w603]
                          tunnel: [w596 sgl[][] []] -> w587
                          tunnel: w579 -> [w597 w606]
                          tunnel: [w597 w606] -> w586
                          tunnel: w578 -> [w595 w605]
                          tunnel: [w595 sgl[] []] -> w585
                          frame False {
                          }
                          frame True {
                            # "Write to disk every f samples (i.e. 1 s intervals)"
                            n172 = Transpose 2D Array(2D array=w603) -> (transposed array=w602:sgl[][])
                            n173 = Build Array (concatenate)(w605, w602) -> (w601:sgl[][])
                            n174 = Transpose 2D Array(2D array=w601) -> (transposed array=w600:sgl[][])
                            n175 = Array To Spreadsheet String(delimiter (Tab)="\t", array=w600, 3:"%.6f" ("format string")) -> (spreadsheet string=w614:string)
                            n176 = Write to Text File(file (use dialog)=w611, text=w614, error in=w610) -> (refnum out=w608:refnum<file>, error out=w609:errorcluster)  [unwired: 1 in, 1 out]
                          }
                        }
                      }
                    }
                    n177 = local write "Checksum ok"(w505) -> ()
                    n178 = Index Array(array=w503, index (row)=0) -> (element=w502:sgl[])  [unwired: 1 in]
                  }
                }
              }
            }
            "chk err" <- w402
            "frm err" <- w403
            n179 = Greater Or Equal?(x=w398, y=w399) -> (x >= y?=w400:bool)
            n180 = call <vilib>:"Clear Errors.vi"("error in (no error)"=w408, "specific error code to clear (0: all)"=1073676294) -> ("error out"=w407:errorcluster)  [unwired: 4 in, 1 out]
            n181 = local write "Error"(w407) -> ()
            n182 = Compound Arithmetic op=OR(w407, "Stop Data", w400) -> (w426:bool)
          }
          n183 = case shown="True" w367 {
            tunnel: [w615 w628] -> w377
            tunnel: w372 -> [w615 w620]
            tunnel: w371 -> [_ w621]
            tunnel: w355 -> [_ w619]
            tunnel: w354 -> [_ w618]
            frame False {
            }
            frame True {
              # "Write any remaining data to disk, then close file"
              n184 = Transpose 2D Array(2D array=w619) -> (transposed array=w625:sgl[][])
              n185 = Build Array (concatenate)(w618, w625) -> (w626:sgl[][])
              n186 = Transpose 2D Array(2D array=w626) -> (transposed array=w627:sgl[][])
              n187 = Array To Spreadsheet String(delimiter (Tab)="\t", array=w627, 3:"%.6f" ("format string")) -> (spreadsheet string=w622:string)
              n188 = Write to Text File(file (use dialog)=w621, text=w622, error in=w620) -> (refnum out=w617:refnum<file>, error out=w616:errorcluster)  [unwired: 1 in, 1 out]
              n189 = Close File(refnum=w617, error in=w616) -> (error out=w628:errorcluster)  [unwired: 1 out]
            }
          }
          n190 = Transpose 2D Array(2D array=w342) -> (transposed array=w345:sgl[][])
          n191 = Transpose 2D Array(2D array=w336) -> (transposed array=w344:sgl[][])
          n192 = Transpose 2D Array(2D array=w335) -> (transposed array=w343:sgl[][])
          n193 = Multiply(x=w346, y=sgl 2000.0) -> (x*y=w358:sgl)
          n194 = To Unsigned Long Integer(number=w358) -> (unsigned 32bit integer=w356:u32)
          n195 = Build Array (concatenate)(w345, w341, w340, w339, w338, w337, w344, w343) -> (w334:sgl[][])
          n196 = call "8HP_Send Cmd.vi"("Operation"=T2 "d" ("Combo Box"), "Port"=w364) -> ("Error Out"=w361:errorcluster, "Port out"=w362:refnum<visa-resource-name>)  [unwired: 2 in]
          n197 = call "Clear buffer.vi"("Error in"=w361, "dt for timeout (ms)"=w356, "VISA resource name in"=w362) -> ("Error out"=w359:errorcluster, "VISA resource name out"=w360:refnum<visa-resource-name>)  [unwired: 3 in]
          n198 = call "Close serial port.vi"("Error in"=w359, "VISA resource name"=w360) -> ("Error out"=w378:errorcluster)  [unwired: 9 in]
        }
      }
      n199 = local write "Stream enabled"(w268) -> ()
      n200 = Merge Errors(w265, w266, w260) -> (w264:errorcluster)
    }
    frame "d" {
      # "Disable USB streaming"
      n201 = flat-sequence {
        tunnel: [w641] -> w634
        tunnel: w633 -> [w641]
        tunnel: w629 -> [w640]
        tunnel: [w635] -> w630
        tunnel: w634 -> [w650]
        tunnel: [w649] -> w632
        tunnel: [TRUE] -> w631
        tunnel: w630 -> [w643]
        frame #0 {
          n202 = Reciprocal(x=w640) -> (1/x=w639:dbl)
          n203 = disable-structure shown="Disabled" {
            frame Disabled {
              n204 = local write "Main"(T1."Data stream" ("Main")) -> ()
            }
            frame Enabled {
            }
          }
          n205 = To Single Precision Float(number=w639) -> (single precision float=w636:sgl)
          n206 = Multiply(x=w636, y=sgl 2000.0) -> (x*y=w637:sgl)
          n207 = To Unsigned Long Integer(number=w637) -> (unsigned 32bit integer=w635:u32)
        }
        frame #1 {
          n208 = local read "COM port"() -> (w651:refnum<visa-resource-name>)
          n209 = call "Open serial port.vi"("timeout (ms)"=u32 5000, "VISA resource name"=w651) -> ("Error out"=w652:errorcluster, "VISA resource name out"=w653:refnum<visa-resource-name>)  [unwired: 8 in]
          n210 = call "8HP_Send Cmd.vi"("Error In"=w652, "Operation"=w650, "Port"=w653) -> ("Error Out"=w647:errorcluster, "Port out"=w645:refnum<visa-resource-name>)  [unwired: 1 in]
          n211 = call "Clear buffer.vi"("Error in"=w647, "dt for timeout (ms)"=w643, "VISA resource name in"=w645) -> ("Error out"=w646:errorcluster, "VISA resource name out"=w644:refnum<visa-resource-name>)  [unwired: 3 in]
          n212 = call "Close serial port.vi"("Error in"=w646, "VISA resource name"=w644) -> ("Error out"=w649:errorcluster)  [unwired: 9 in]
        }
      }
    }
    frame "F" {
      # "Set data rate"
      n213 = flat-sequence {
        tunnel: w661 -> [w664]
        tunnel: [w664] -> w660
        tunnel: w660 -> [w671]
        tunnel: [w670] -> w659
        tunnel: [w669] -> w658
        tunnel: [w709] -> w657
        tunnel: w659 -> [w709]
        tunnel: w658 -> [w707]
        tunnel: [w707] -> w656
        tunnel: [TRUE] -> w655
        frame #0 {
          n214 = local write "Returned data rate (Hz)"(u16 0 ("Returned data rate (Hz)")) -> ()
          n215 = local write "received"(FALSE ("sent")) -> ()
          n216 = local write "Main"(T1."Data rate" ("Main")) -> ()
          n217 = local write "sent"(FALSE ("sent")) -> ()
        }
        frame #1 {
          # "to LE"
          n218 = local read "Set data rate (Hz)"() -> (w667:u8)
          n219 = case shown="14, Default" w667 {
            tunnel: [1.0 2.0 4.0 5.0 8.0 10.0 16.0 20.0 25.0 32.0 40.0 50.0 64.0 80.0 100.0 125.0 160.0 200.0 250.0 320.0 400.0 500.0 625.0 800.0 1000.0] -> w670
            frame 0 {
            }
            frame 1 {
            }
            frame 2 {
            }
            frame 3 {
            }
            frame 4 {
            }
            frame 5 {
            }
            frame 6 {
            }
            frame 7 {
            }
            frame 8 {
            }
            frame 9 {
            }
            frame 10 {
            }
            frame 11 {
            }
            frame 12 {
            }
            frame 13 {
            }
            frame 14, Default {
            }
            frame 15 {
            }
            frame 16 {
            }
            frame 17 {
            }
            frame 18 {
            }
            frame 19 {
            }
            frame 20 {
            }
            frame 21 {
            }
            frame 22 {
            }
            frame 23 {
            }
            frame 24 {
            }
          }
          n220 = local read "COM port"() -> (w674:refnum<visa-resource-name>)
          n221 = To Unsigned Word Integer(number=w670) -> (unsigned 16bit integer=w678:u16)
          n222 = Type Cast(type="", x=w678) -> (*(type *) &x=w680:string)
          n223 = call "Open serial port.vi"("timeout (ms)"=u32 5000, "VISA resource name"=w674) -> ("Error out"=w675:errorcluster, "VISA resource name out"=w676:refnum<visa-resource-name>)  [unwired: 8 in]
          n224 = Reverse String(1:w680) -> (0:w668:string)
          n225 = call "8HP_Send Cmd + Data.vi"("Error In"=w675, "Data"=w668, "Operation"=w671, "Port"=w676) -> ("Error Out"=w672:errorcluster, "Port out"=w673:refnum<visa-resource-name>)  [unwired: 1 in]
          n226 = call "Close serial port.vi"("Error in"=w672, "VISA resource name"=w673) -> ("Error out"=w669:errorcluster)  [unwired: 9 in]
        }
        frame #2 {
          n227 = Unbundle By Name(w707) -> ("status"=w708:bool)
          n228 = Not(x=w708) -> (.not. x?=→"sent":bool)
        }
      }
    }
    frame "f" {
      # "Get data rate"
      n229 = flat-sequence {
        tunnel: w717 -> [w720]
        tunnel: [w720] -> w716
        tunnel: w716 -> [w730]
        tunnel: [w733] -> w715
        tunnel: [w735] -> w714
        tunnel: [w742] -> w713
        tunnel: w715 -> [w742]
        tunnel: w714 -> [w740]
        tunnel: [w740] -> w712
        tunnel: [TRUE] -> w711
        frame #0 {
          n230 = local write "received"(FALSE ("sent")) -> ()
          n231 = local write "Main"(T1."Data rate" ("Main")) -> ()
          n232 = local write "sent"(FALSE ("sent")) -> ()
        }
        frame #1 {
          # "to BE"
          n233 = local read "COM port"() -> (w736:refnum<visa-resource-name>)
          n234 = call "Open serial port.vi"("timeout (ms)"=u32 5000, "VISA resource name"=w736) -> ("Error out"=w731:errorcluster, "VISA resource name out"=w732:refnum<visa-resource-name>)  [unwired: 8 in]
          n235 = call "8HP_Send Cmd.vi"("Error In"=w731, "Operation"=w730, "Port"=w732) -> ("Error Out"=w728:errorcluster, "Port out"=w727:refnum<visa-resource-name>)  [unwired: 1 in]
          n236 = VISA Read(VISA resource name=w727, byte count=u32 2, error in (no error)=w728) -> (VISA resource name out=w725:refnum<visa-resource-name>, read buffer=w724:string, error out=w726:errorcluster)  [unwired: 1 out]
          n237 = Reverse String(1:w724) -> (0:w734:string)
          n238 = call "Close serial port.vi"("Error in"=w726, "VISA resource name"=w725) -> ("Error out"=w735:errorcluster)  [unwired: 9 in]
          n239 = Type Cast(type=u16 0 ("byte count"), x=w734) -> (*(type *) &x=w722:u16)
          "Returned data rate (Hz)" <- w722
          n240 = To Double Precision Float(number=w722) -> (double precision float=w733:dbl)
        }
        frame #2 {
          n241 = Unbundle By Name(w740) -> ("status"=w741:bool)
          n242 = Not(x=w741) -> (.not. x?=→"received":bool)
        }
      }
    }
    frame "N" {
      # "Get serial number"
      n243 = flat-sequence {
        tunnel: w746 -> [w750]
        tunnel: [w750] -> w745
        tunnel: [TRUE] -> w747
        tunnel: w745 -> [w756]
        tunnel: [w755] -> w744
        frame #0 {
          n244 = local write "Main"(T1."Action" ("Main")) -> ()
          "Serial number" <- sgl 0.0 ("Numeric")
        }
        frame #1 {
          # "to BE"
          n245 = local read "COM port"() -> (w757:refnum<visa-resource-name>)
          n246 = call "Open serial port.vi"("timeout (ms)"=u32 5000, "VISA resource name"=w757) -> ("Error out"=w764:errorcluster, "VISA resource name out"=w765:refnum<visa-resource-name>)  [unwired: 8 in]
          n247 = call "8HP_Send Cmd.vi"("Error In"=w764, "Operation"=w756, "Port"=w765) -> ("Error Out"=w762:errorcluster, "Port out"=w763:refnum<visa-resource-name>)  [unwired: 1 in]
          n248 = VISA Read(VISA resource name=w763, byte count=u32 4, error in (no error)=w762) -> (VISA resource name out=w760:refnum<visa-resource-name>, read buffer=w752:string, error out=w759:errorcluster)  [unwired: 1 out]
          n249 = call "Close serial port.vi"("Error in"=w759, "VISA resource name"=w760) -> ("Error out"=w755:errorcluster)  [unwired: 9 in]
          n250 = Reverse String(1:w752) -> (0:w753:string)
          n251 = Type Cast(type=sgl 0.0 ("byte count"), x=w753) -> (*(type *) &x=w751:sgl)
          n252 = local write "Serial number"(w751) -> ()
        }
      }
    }
    frame "X" {
      # "Exit"
    }
    frame Default {
    }
  }
  "All samples out" <- w3
  n253 = Merge Errors(w10, w9) -> (w8:errorcluster)
  n254 = call <vilib>:"Clear Errors.vi"("error in (no error)"=w8, "specific error code to clear (0: all)"=1073676294) -> ("error out"=w1:errorcluster)  [unwired: 4 in, 1 out]
  "Error" <- w1
  n255 = local write "Error"(w1) -> ()
